vi "LHF.DB.Mongo.Collection.FindOne.vi"(8 "error in (no error)":errorcluster, 9 "query":refnum<k24>, 10 "Collection":string, 11 "LHF.DB.Mongo in":refnum<class "LHF.DB.Mongo.lvclass">) -> (0 "error out":errorcluster, 2 "Document":string, 3 "LHF.DB.Mongo out":refnum<class "LHF.DB.Mongo.lvclass">, 5 "ObjectID":string)   [LabVIEW 2013, in "LHF.DB.Mongo.lvclass"]
uses:
  LHF.DB.Mongo.lvclass
  C:/Users/schim/Desktop/Projetos/LabVIEW-MongoDB/src/Driver/MongoDB.Driver.dll
  Driver/MongoDB.Driver.dll
  C:/Users/schim/Desktop/Projetos/LabVIEW-MongoDB/src/Driver/MongoDB.Bson.dll
  Driver/MongoDB.Bson.dll
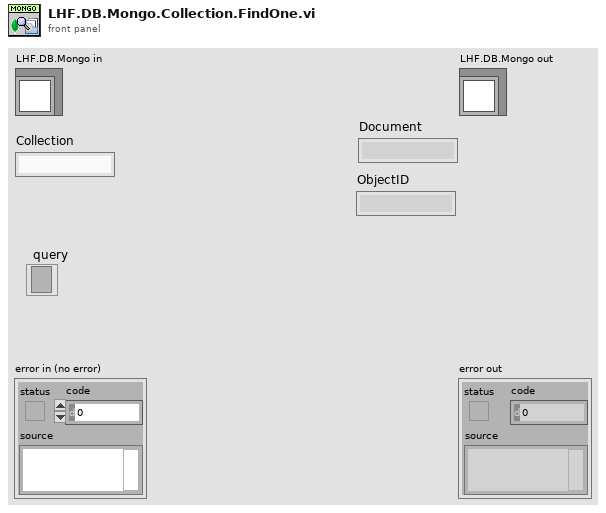
[diagram p1: front panel]
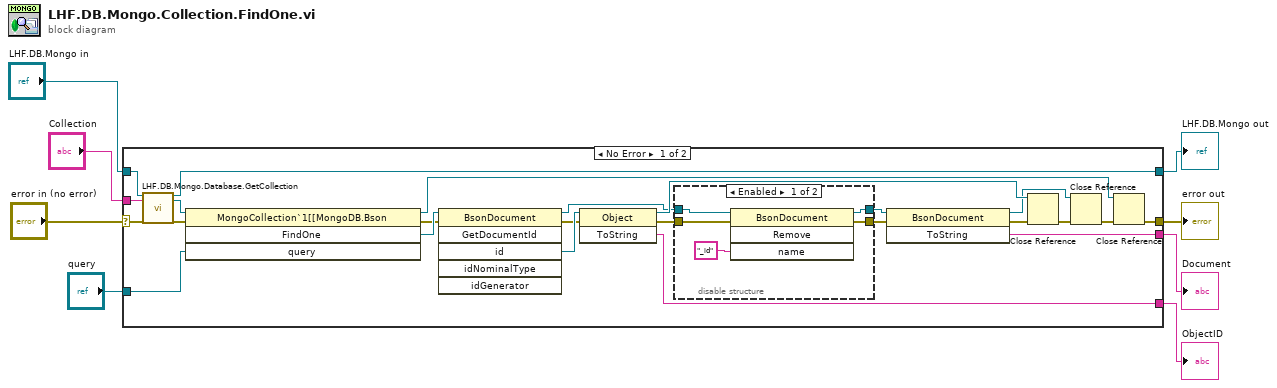
[diagram p0: block diagram]
diagram:
  n1 = case shown="No Error" "error in (no error)" {
    selector: "error in (no error)" -> [w27 w41]
    tunnel: [w29 w41] -> w7
    tunnel: [w31 w40] -> w5
    tunnel: "LHF.DB.Mongo in" -> [w30 w40]
    tunnel: "Collection" -> [w32 _]
    tunnel: "query" -> [w23 _]
    tunnel: [w25 _] -> w2
    tunnel: [w24 _] -> w1
    frame No Error {
      n2 = call "LHF.DB.Mongo.Database.GetCollection.vi"("LHF.DB.Mongo in"=w30, "collectionName"=w32, "error in (no error)"=w27) -> ("LHF.DB.Mongo in"=w31:refnum<class "LHF.DB.Mongo.lvclass">, "MongoCollection"=w28:refnum<k24>, "error out"=w26:errorcluster)  [unwired: 14 in]
      n3 = invoke class="MongoCollection`1[[MongoDB.Bson" method="FindOne"(reference=w28, error in=w26, "query"=w23) -> (reference out=w22:refnum<k24>, error out=w9:errorcluster, "FindOne"=w10:refnum<k24>)  [unwired: 1 in, 1 out]
      n4 = invoke class="BsonDocument" method="GetDocumentId"(reference=w10, error in=w9) -> (reference out=w15:refnum<k24>, error out=w20:errorcluster, "id"=w21:refnum<k24>)  [unwired: 4 in, 3 out]
      n5 = invoke class="Object" method="ToString"(reference=w21, error in=w20) -> (reference out=w18:refnum<k24>, error out=w16:errorcluster, "ToString"=w25:string)  [unwired: 1 in]
      n6 = disable-structure shown="Enabled" {
        disable-tunnel: [w36 w39] -> w17
        disable-tunnel: w16 -> [w35 w38]
        disable-tunnel: w15 -> [w34 w39]
        disable-tunnel: [w33 w38] -> w12
        frame Enabled {
          n7 = invoke class="BsonDocument" method="Remove"(reference=w34, error in=w35, "name"="_id") -> (reference out=w36:refnum<k24>, error out=w33:errorcluster)  [unwired: 1 in, 2 out]
        }
        frame Disabled {
        }
      }
      n8 = invoke class="BsonDocument" method="ToString"(reference=w17, error in=w12) -> (reference out=w14:refnum<k24>, error out=w13:errorcluster, "ToString"=w24:string)  [unwired: 1 in]
      n9 = Close Reference(reference=w18, error in (no error)=w13) -> (error out=w19:errorcluster)
      n10 = Close Reference(reference=w14, error in (no error)=w19) -> (error out=w11:errorcluster)
      n11 = Close Reference(reference=w22, error in (no error)=w11) -> (error out=w29:errorcluster)
    }
    frame Error {
    }
  }
  "error out" <- w7
  "LHF.DB.Mongo out" <- w5
  "Document" <- w1
  "ObjectID" <- w2
